vi "KB-RS232-MessageDealWith.vi"(11 "Receive Message":string) -> (1 "CCD Step Number":i32, 2 "Motion Done":bool, 3 "EMG":bool)   [LabVIEW 2015]
panel:
  out "数组 4":i32[](array[numeric])
  out "数组 3":string[](array[string])
  out "数组 2":string[][](array[string])
  out "x/y":dbl
  out "大小":i32
  out "已删除元素的数组子集":string[](array[string])
  out "数组":string[](array[string])
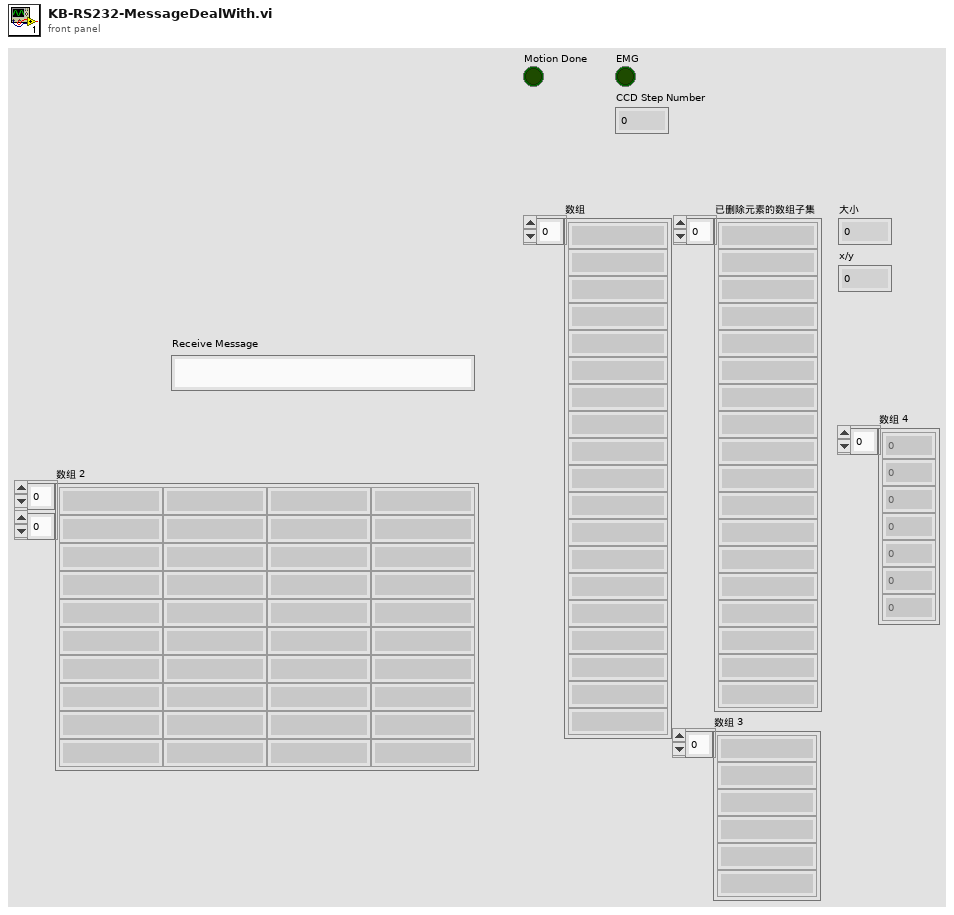
[diagram p1: front panel]
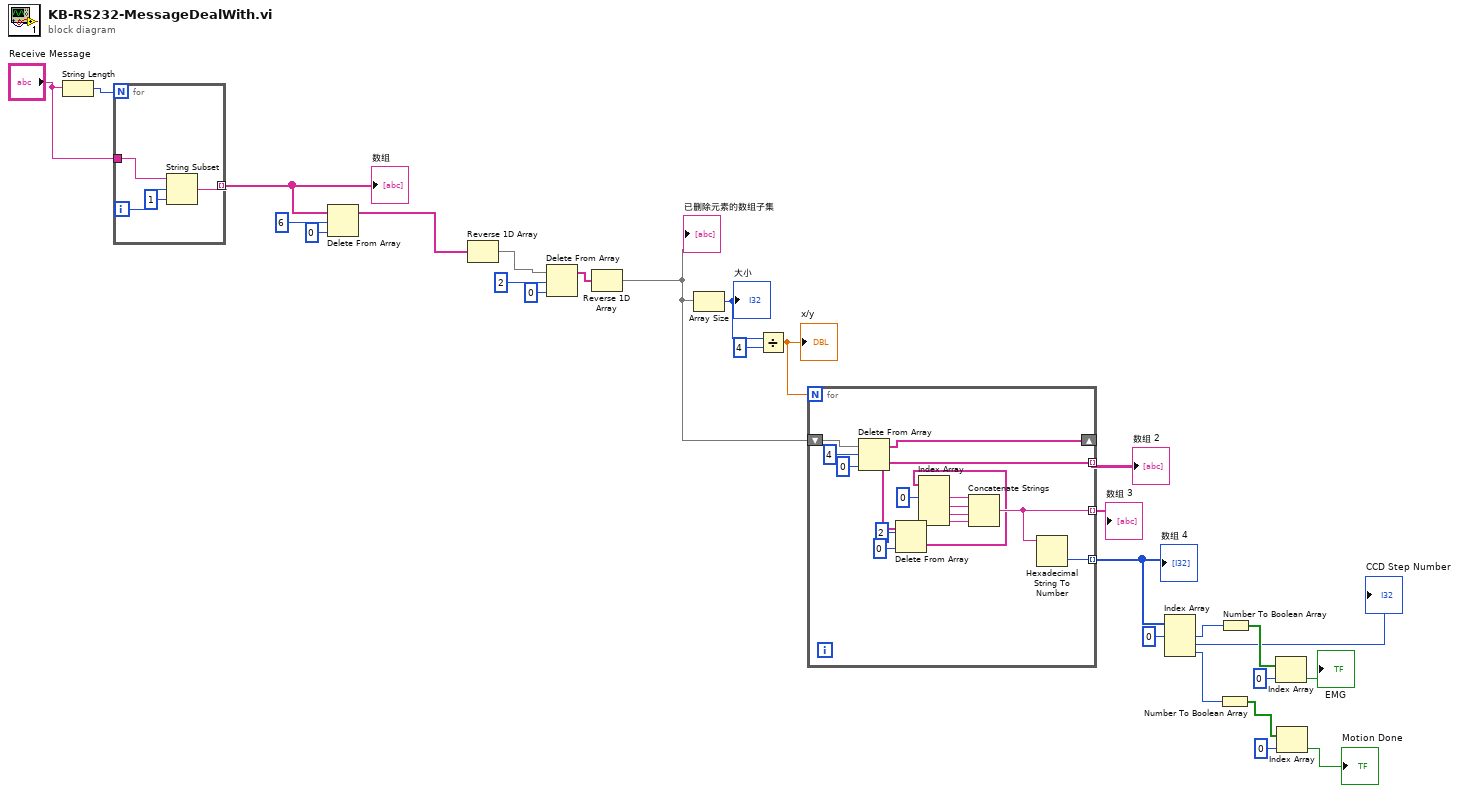
[diagram p0: block diagram]
diagram:
  n1 = String Length(string="Receive Message") -> (length=w27:i32)
  n2 = for {
    N: w27 -> [_]
    tunnel: "Receive Message" -> [w31]
    tunnel: [w28] -> w25 mode=indexing
    i -> [w30]
    n3 = String Subset(string=w31, offset (0)=w30, length (rest)=1 ("长度（剩余）")) -> (substring=w28:string)
  }
  "数组" <- w25
  n4 = Delete From Array(array=w25, length=6 ("长度"), index=0 ("索引")) -> (array with subset deleted=w22:string[])  [unwired: 1 out]
  n5 = Reverse 1D Array(array=w22) -> (reversed array=w19:string[])
  n6 = Delete From Array(array=w19, length=2 ("长度"), index=0 ("索引")) -> (array with subset deleted=w18:string[])  [unwired: 1 out]
  n7 = Reverse 1D Array(array=w18) -> (reversed array=w14:string[])
  "已删除元素的数组子集" <- w14
  n8 = Array Size(array=w14) -> (size(s)=w17:i32)
  "大小" <- w17
  n9 = Divide(x=w17, y=4) -> (x/y=w15:dbl)
  "x/y" <- w15
  n10 = for {
    N: w15 -> [_]
    shift-right: [w43] -> _
    shift-left: w14 -> [w46]
    tunnel: [w35] -> w13 mode=indexing
    tunnel: [w37] -> w12 mode=indexing
    tunnel: [w36] -> w11 mode=indexing
    n11 = Delete From Array(array=w46, length=4 ("长度"), index=0 ("索引")) -> (deleted portion=w35:string[], array with subset deleted=w43:string[])
    n12 = Delete From Array(array=w35, length=2 ("长度"), index=0 ("索引")) -> (deleted portion=w32:string[])  [unwired: 1 out]
    n13 = Index Array(array=w32, index #1=0 ("索引")) -> (element #1=w41:string, element #2=w40:string, element #3=w39:string, element #4=w38:string)  [unwired: 3 in]
    n14 = Concatenate Strings(w41, w40, w39, w38) -> (w37:string)
    n15 = Hexadecimal String To Number(string=w37) -> (number=w36:u32)  [unwired: 2 in, 1 out]
  }
  "数组 2" <- w13
  "数组 3" <- w12
  "数组 4" <- w11
  n16 = Index Array(array=w11, index #1=0 ("索引")) -> (element #1=w9:u32, element #2=→"CCD Step Number":u32, element #3=w4:u32)  [unwired: 2 in]
  n17 = Number To Boolean Array(number=w4) -> (Boolean array=w2:bool[])
  n18 = Number To Boolean Array(number=w9) -> (Boolean array=w8:bool[])
  n19 = Index Array(array=w8, index=0 ("索引")) -> (element=→"EMG":bool)
  n20 = Index Array(array=w2, index=0 ("索引")) -> (element=→"Motion Done":bool)
